vi "DB Check.vi"(8 "error in":errorcluster, 9 "DB":T1, 10 "SQL query":string, 11 "Database in":refnum<class "Database.lvclass">) -> (0 "error out":errorcluster, 2 "data":string[][](array[string]), 3 "Database out":refnum<class "Database.lvclass">)   [LabVIEW 2023, in "HardwareAbstractionLayer_LVOOP.lvlib" / "Database.lvclass"]
uses:
  Database.lvclass
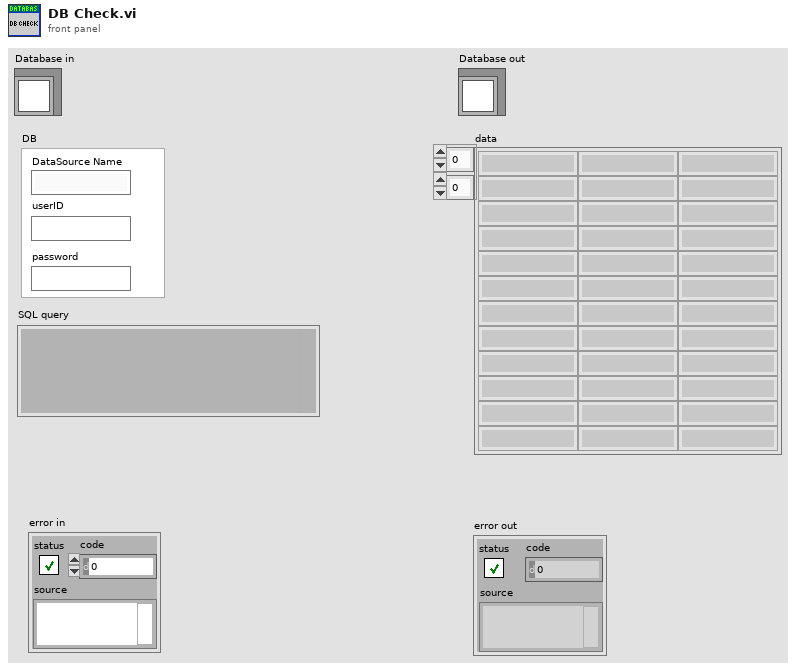
[diagram p1: front panel]
types:
  T1 = cluster{"DataSource Name":string, "userID":string, "password":string}
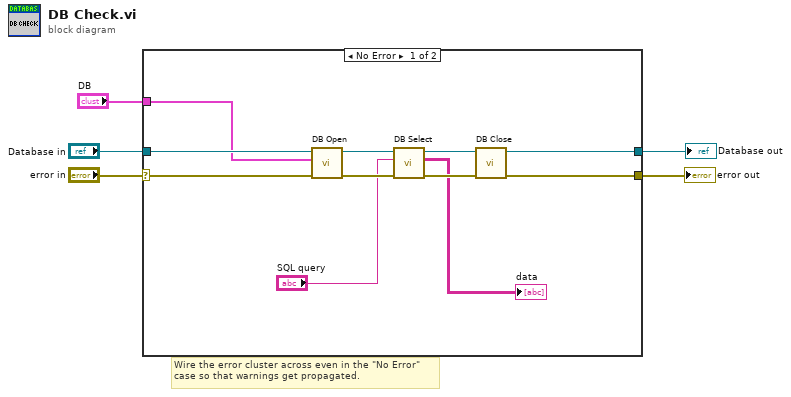
[diagram p0: block diagram]
diagram:
  # "Wire the error cluster across even in the \"No Error\"\ncase so that warnings get propagated."
  n1 = case shown="No Error" "error in" {
    selector: "error in" -> [w13 w18]
    tunnel: [w12 w18] -> w4
    tunnel: [w9 w17] -> w2
    tunnel: "Database in" -> [w16 w17]
    tunnel: "DB" -> [w6 _]
    frame No Error {
      n2 = call-dynamic "DB Open.vi"("error in"=w13, "DB"=w6, "Database in"=w16) -> ("error out"=w10:errorcluster, "Database out"=w15:refnum<class "Database.lvclass">)  [unwired: 7 in]
      n3 = call-dynamic "DB Select.vi"("error in (no error)"=w10, "SQL query"="SQL query", "Database in"=w15) -> ("error out"=w11:errorcluster, "data"=→"data":string[][], "Database out"=w14:refnum<class "Database.lvclass">)  [unwired: 6 in]
      n4 = call-dynamic "DB Close.vi"("error in"=w11, "Database in"=w14) -> ("error out"=w12:errorcluster, "Database out"=w9:refnum<class "Database.lvclass">)  [unwired: 8 in]
    }
    frame Error {
    }
  }
  "error out" <- w4
  "Database out" <- w2
